vi "PushIncons.vi"(10 "node ref in":refnum<data-value>, 11 "RVCLibrary_Bug in":refnum<class "RVCLibrary_Bug2.lvclass">) -> (2 "node ref out":refnum<data-value>, 3 "RVCLibrary_Bug out":refnum<class "RVCLibrary_Bug2.lvclass">)   [LabVIEW 2013, in "RVCLibrary_Bug2.lvclass"]
uses:
  RVCLibrary_Bug2.lvclass
  <vilib>/robotics/Navigation/shared/MapNode/AbstractDstarNode/NI_Robotics_AbstractDstarNode.lvclass
  RVCLibrary_Bug2.lvclass/RVCLibrary_Bug2.ctl
  <vilib>/robotics/Navigation/shared/InconsistentList/NI_Robotics_InconsistentList.lvclass
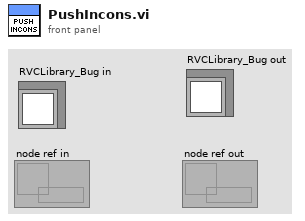
[diagram p1: front panel]
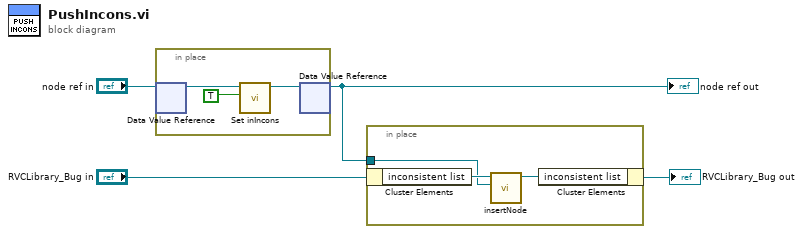
[diagram p0: block diagram]
diagram:
  n1 = in-place {
    n2 = in-place-dvr #1("node ref in") -> (w7:refnum<class "NI_Robotics_AbstractDstarNode.lvclass">)  [unwired: 1 out]
    n3 = call <vilib>:"Set inIncons.vi"("inIncons"=TRUE, "AbstractDstarNode in"=w7) -> ("AbstractDstarNode out"=w6:refnum<class "NI_Robotics_AbstractDstarNode.lvclass">)  [unwired: 9 in]
    n4 = in-place-dvr #1(w6) -> (w3:refnum<data-value>)  [unwired: 1 out]
  }
  "node ref out" <- w3
  n5 = in-place {
    in-place-border: w3 -> [w8]
    n6 = in-place-cluster #2("RVCLibrary_Bug in") -> ("inconsistent list"=w10:refnum<class "NI_Robotics_InconsistentList.lvclass">)
    n7 = call <vilib>:"insertNode.vi"("node ref in"=w8, "InconsistentList in"=w10) -> ("InconsistentList out"=w9:refnum<class "NI_Robotics_InconsistentList.lvclass">)  [unwired: 8 in, 1 out]
    n8 = in-place-cluster #2("inconsistent list"=w9) -> (→"RVCLibrary_Bug out":refnum<class "RVCLibrary_Bug2.lvclass">)
  }
